vi "ReadTCPIPPort.vi"(8 "error in (no error)":errorcluster, 11 "TCP Network Connection in":refnum<k5>) -> (0 "error out":errorcluster, 2 "data out":string, 3 "TCP Network Connection out":refnum<k5>)   [LabVIEW 2020]
uses:
  <vilib>/Utility/error.llb/Trim Whitespace One-Sided.vi
panel:
  # "Input"
  # "Output"
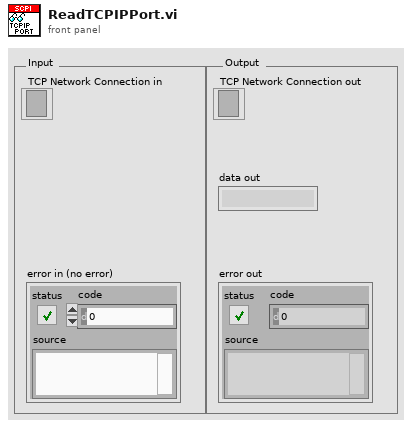
[diagram p1: front panel]
types:
  T1 = enum16{"Standard", "Buffered", "CRLF", "Immediate"}
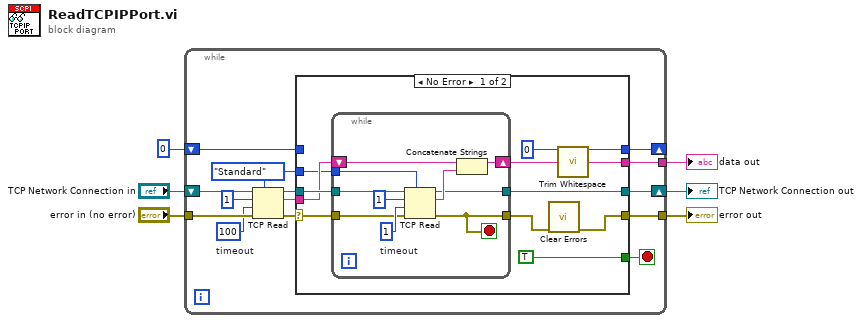
[diagram p0: block diagram]
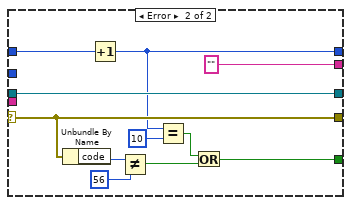
[diagram p2: hidden frame]
diagram:
  n1 = while {
    tunnel: [w11] -> w5
    shift-right: [w13] -> w3
    shift-left: "TCP Network Connection in" -> [w20]
    tunnel: "error in (no error)" -> [w19]
    tunnel: [w12] -> w4
    shift-right: [w8] -> _
    shift-left: 0 -> [w9]
    stop <- w10 stop-if-true
    w7 = T1."Standard" ("mode (standard)")
    w18 = 100  # timeout
    n2 = TCP Read(connection ID=w20, bytes to read=1, error in (no error)=w19, 7:w7, 9:w18) -> (connection ID out=w14:refnum<k5>, data out=w15:string, error out=w16:errorcluster)
    n3 = case shown="No Error" w16 {
      selector: w16 -> [w31 w50]
      tunnel: w15 -> [w29 _]
      tunnel: w14 -> [w30 w51]
      tunnel: [w28 w51] -> w13
      tunnel: [w22 w50] -> w12
      tunnel: [w21 "" ("data out")] -> w11
      tunnel: [TRUE w46] -> w10
      tunnel: w9 -> [_ w45]
      tunnel: [0 w43] -> w8
      tunnel: w7 -> [w24 _]
      frame No Error {
        n4 = while {
          tunnel: w31 -> [w39]
          tunnel: w30 -> [w38]
          shift-right: [w37] -> w27
          shift-left: w29 -> [w36]
          tunnel: [w34] -> w28
          tunnel: [w33] -> w23
          tunnel: w24 -> [w32]
          stop <- w33 stop-if-true
          w40 = 1  # timeout
          n5 = TCP Read(connection ID=w38, bytes to read=1, error in (no error)=w39, 7:w32, 9:w40) -> (connection ID out=w34:refnum<k5>, data out=w35:string, error out=w33:errorcluster)
          n6 = Concatenate Strings(w36, w35) -> (w37:string)
        }
        n7 = call <vilib>:"Clear Errors.vi"("error in (no error)"=w23) -> ("error out"=w22:errorcluster)  [unwired: 5 in, 1 out]
        n8 = call <vilib>:"Trim Whitespace.vi"("string"=w27) -> ("trimmed string"=w21:string)  [unwired: 1 in]
      }
      frame Error {
        n9 = Unbundle By Name(w50) -> ("code"=w49:i32)
        n10 = Increment(x=w45) -> (x+1=w43:i32)
        n11 = Not Equal?(x=w49, y=56) -> (x != y?=w47:bool)
        n12 = Equal?(x=w43, y=10) -> (x = y?=w44:bool)
        n13 = Or(x=w44, y=w47) -> (x .or. y?=w46:bool)
      }
    }
  }
  "data out" <- w5
  "error out" <- w4
  "TCP Network Connection out" <- w3
